vi "FlexDDS-NG_DCP_Wait_BNC.vi"(9 "Trigger":T1(ring), 10 "Channels":T2(ring), 11 "appended instruction string in":string) -> (3 "appended instruction string":string)   [LabVIEW 2010]
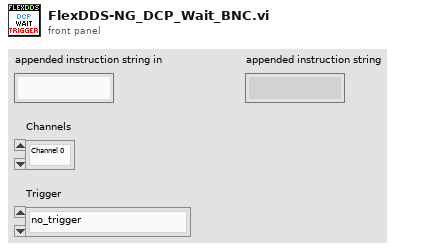
[diagram p1: front panel]
types:
  T1 = enum16{"no_trigger", "BNC_IN_A_RISING", "BNC_IN_A_FALLING", "BNC_IN_B_RISING", "BNC_IN_B_FALLING", "BNC_IN_C_RISING", "BNC_IN_C_FALLING"}
  T2 = enum32{"Channel 0", "Channel 1", "Both channels"}
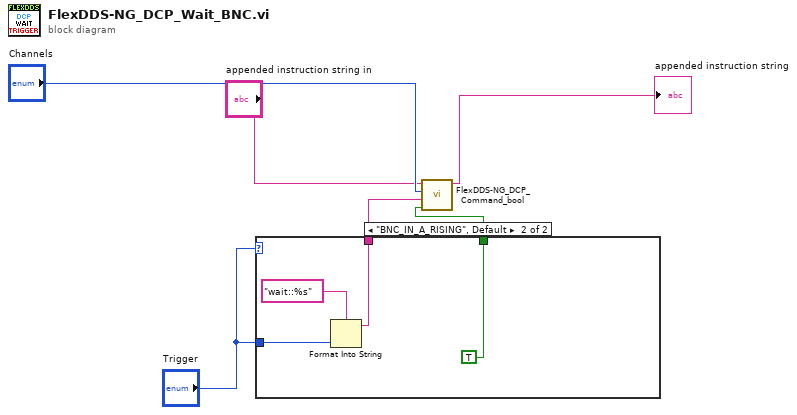
[diagram p0: block diagram]
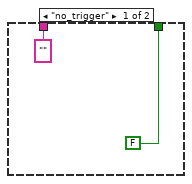
[diagram p2: hidden frame]
diagram:
  n1 = case shown="\"BNC_IN_A_RISING\", Default" "Trigger" {
    tunnel: "Trigger" -> [_ w12]
    tunnel: [FALSE TRUE] -> w5
    tunnel: ["" w9] -> w6
    frame "no_trigger" {
    }
    frame "BNC_IN_A_RISING", Default {
      n2 = Format Into String(format string="wait::%s", w12) -> (resulting string=w9:string)  [unwired: 2 in, 1 out]
    }
  }
  n3 = call "FlexDDS-NG_DCP_Command_bool.vi"("Write DCP command?"=w5, "command string"=w6, "Channels"="Channels", "initial instruction string"="appended instruction string in") -> ("appended instruction string"=→"appended instruction string":string)  [unwired: 7 in]
